vi "Generate Response Body.vi"(10 "Body":string, 11 "HEADIN":string) -> (3 "MessageOUT":string)   [LabVIEW 2019, in "HTTP Server.lvlib"]
uses:
  HTTP Server.lvlib
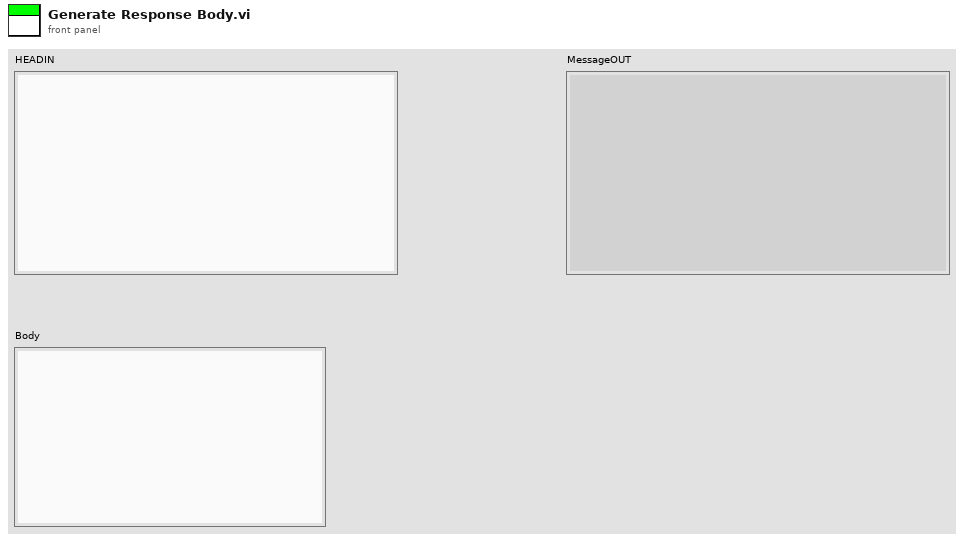
[diagram p1: front panel]
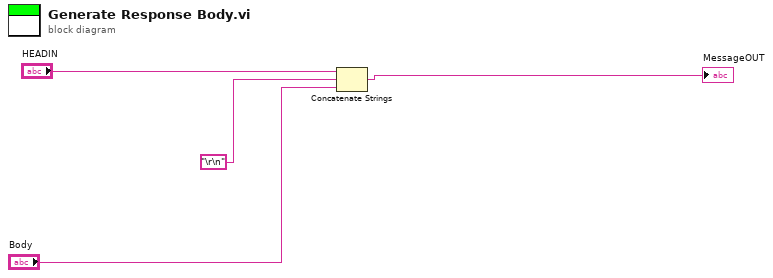
[diagram p0: block diagram]
diagram:
  n1 = Concatenate Strings("HEADIN", "\r\n", "Body") -> (→"MessageOUT":string)
